vi "CRC_add.vi"(8 "error in (no error)":errorcluster, 11 "ISO 15693 DOWN in":refnum<class "ISO 15693 DOWN.lvclass">) -> (0 "error out":errorcluster, 3 "ISO 15693 DOWN out":refnum<class "ISO 15693 DOWN.lvclass">)   [LabVIEW 2019, in "ISO 15693 DOWN.lvclass"]
uses:
  ISO 15693 DOWN.lvclass
  TypeDef/Store.ctl
  ISO 15693 DOWN.lvclass/ISO 15693 DOWN.ctl
  Libraries/CRC/CRC16CITT_B_15.vi
  RFID system.lvclass
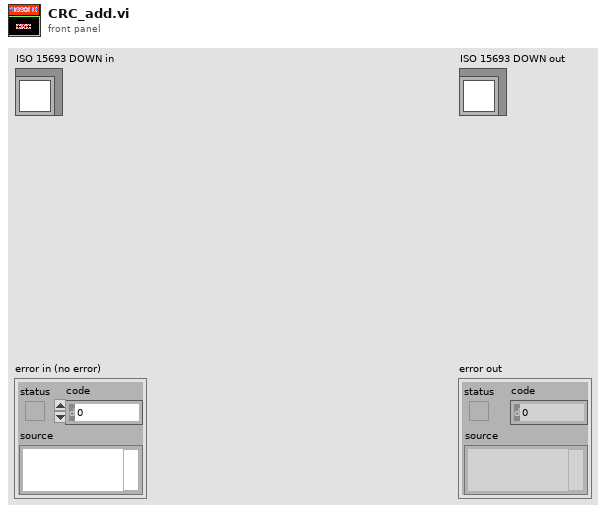
[diagram p1: front panel]
types:
  T1 = typedef "Store.ctl" = enum16{"envelope", "noise", "demSubCar", "CH_frame", "Decode", "demodulate", "in", "out", "sum", "subCarrier", "frame", "command", "encode", "modulate", "encode_UP", "modulate_up", "demod_up", "envelop_up", "sum_up", "out_up", "in_up"}
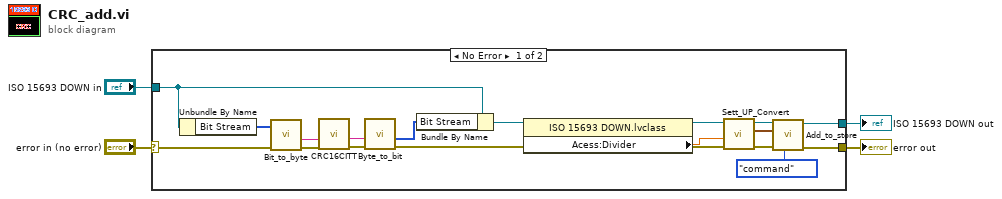
[diagram p0: block diagram]
diagram:
  n1 = case shown="No Error" "error in (no error)" {
    selector: "error in (no error)" -> [w11 w23]
    tunnel: [w15 w23] -> w3
    tunnel: "ISO 15693 DOWN in" -> [w18 w24]
    tunnel: [w19 w24] -> w1
    frame No Error {
      n2 = Unbundle By Name(w18) -> ("Bit Stream"=w14:u8[])
      n3 = call "Bit_to_byte.vi"("Error In"=w11, "Array of bit"=w14) -> ("Error Out"=w9:errorcluster, "BYTE"=w10:string)  [unwired: 7 in, 1 out]
      n4 = call-poly "CRC16CITT.vi"("Error In"=w9, "DATA PACKET"=w10) -> ("Error Out"=w8:errorcluster, "DATA PACKET+CRC"=w7:string)  [unwired: 7 in, 1 out]
      n5 = call "Byte_to_bit.vi"("Error In"=w8, "BYTE"=w7) -> ("Error Out"=w12:errorcluster, "Arrray of bit (str)"=w13:u8[])  [unwired: 5 in, 1 out]
      n6 = Bundle By Name(cluster=w18, "Bit Stream"=w13) -> (w17:refnum<class "ISO 15693 DOWN.lvclass">)
      n7 = property class="ISO 15693 DOWN.lvclass"(reference=w17) -> (reference out=w6:refnum<class "ISO 15693 DOWN.lvclass">, "Acess:Divider"=w5:dbl)  [unwired: 1 in, 1 out]
      n8 = call-dynamic "Sett_UP_Convert.vi"("error in (no error)"=w12, "Divider(1)"=w5, "ISO 15693 DOWN in"=w6) -> ("error out"=w20:errorcluster, "Waveform"=w21:waveform(dbl), "ISO 15693 DOWN out"=w22:refnum<class "ISO 15693 DOWN.lvclass">)  [unwired: 6 in]
      n9 = call "Add_to_store.vi"("Store"=Store."command", "error in (no error)"=w20, "Waveform"=w21, "RFID system in"=w22) -> ("error out"=w15:errorcluster, "RFID system out"=w19:refnum<class "ISO 15693 DOWN.lvclass">)  [unwired: 6 in]
    }
    frame Error {
    }
  }
  "error out" <- w3
  "ISO 15693 DOWN out" <- w1
